vi "ApplyVIPC.vi"   [LabVIEW 2021]
uses:
  <vilib>/Wiresmith Technology/G CLI/CLI Class/CLI.lvclass
  <vilib>/JKI/VIPM API/VIPM API_vipm_api.lvlib
types:
  T1 = enum32{"Invalid", "Standard", "Closed", "Hidden", "Minimized", "Maximized"}
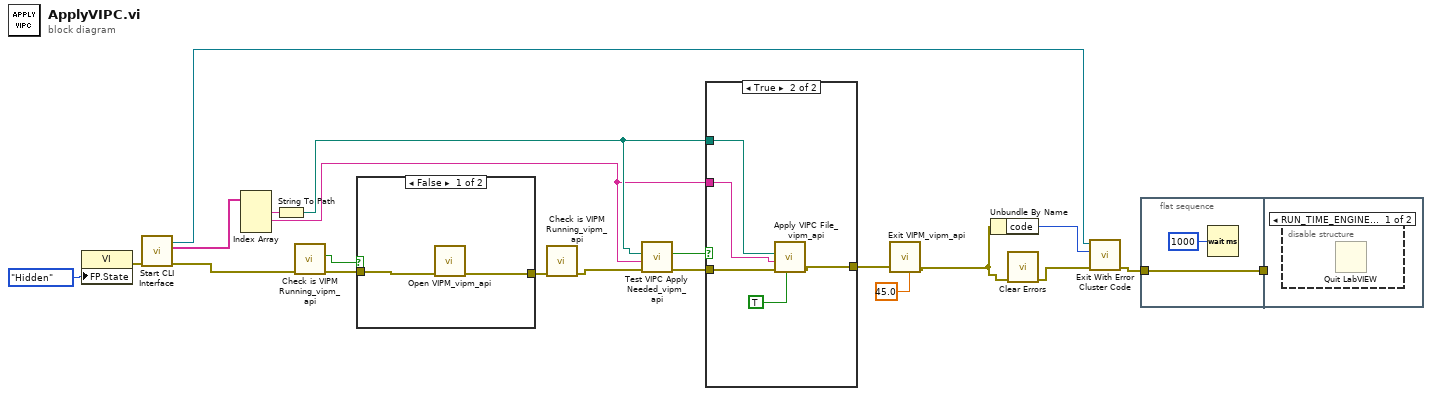
[diagram p0: block diagram]
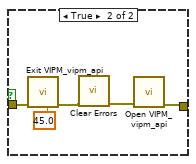
[diagram p2: hidden frame]
diagram:
  n1 = property class="VI"("FP.State"=T1."Hidden" ("Front Panel Window:State")) -> (error out=w20:errorcluster)  [unwired: 2 in, 1 out]
  n2 = call <vilib>:"Start CLI Interface.vi"("error in (no error)"=w20) -> ("error out"=w4:errorcluster, "Custom Parameters"=w18:string[], "CLI out"=w19:refnum<class "CLI.lvclass">)  [unwired: 7 in, 1 out]
  n3 = Index Array(array=w18) -> (element #1=w15:string, element #2=w11:string)  [unwired: 3 in, 1 out]
  n4 = String To Path(string=w15) -> (path=w12:path)
  n5 = call <vilib>:"Check is VIPM Running_vipm_api.vi"("error in (no error)"=w4) -> ("error out"=w10:errorcluster, "is Running"=w9:bool)  [unwired: 9 in]
  n6 = case shown="False" w9 {
    tunnel: w10 -> [w23 w28]
    tunnel: [w22 w24] -> w8
    frame False {
      n7 = call <vilib>:"Open VIPM_vipm_api.vi"("error in (no error)"=w23) -> ("error out"=w22:errorcluster)  [unwired: 10 in]
    }
    frame True {
      n8 = call <vilib>:"Exit VIPM_vipm_api.vi"("Timeout in seconds (0: no timeout)"=45.0, "error in (no error)"=w28) -> ("error out"=w27:errorcluster)  [unwired: 9 in]
      n9 = call <vilib>:"Clear Errors.vi"("error in (no error)"=w27) -> ("error out"=w25:errorcluster)  [unwired: 5 in, 1 out]
      n10 = call <vilib>:"Open VIPM_vipm_api.vi"("error in (no error)"=w25) -> ("error out"=w24:errorcluster)  [unwired: 10 in]
    }
  }
  n11 = call <vilib>:"Check is VIPM Running_vipm_api.vi"("error in (no error)"=w8) -> ("error out"=w5:errorcluster)  [unwired: 9 in, 1 out]
  n12 = call <vilib>:"Test VIPC Apply Needed_vipm_api.vi"("error in (no error)"=w5, "LabVIEW Version (use vipc version)"=w11, "VIPC File Path"=w12) -> ("error out"=w13:errorcluster, "Need to Apply?"=w14:bool)  [unwired: 6 in, 1 out]
  n13 = case shown="True" w14 {
    tunnel: w13 -> [w29 w33]
    tunnel: [w29 w32] -> w6
    tunnel: w12 -> [_ w31]
    tunnel: w11 -> [_ w30]
    frame False {
    }
    frame True {
      n14 = call <vilib>:"Apply VIPC File_vipm_api.vi"("quiet? (T)"=TRUE, "error in (no error)"=w33, "LabVIEW Version"=w30, "VIPC File"=w31) -> ("error out"=w32:errorcluster)  [unwired: 7 in]
    }
  }
  n15 = call <vilib>:"Exit VIPM_vipm_api.vi"("Timeout in seconds (0: no timeout)"=45.0, "error in (no error)"=w6) -> ("error out"=w2:errorcluster)  [unwired: 9 in]
  n16 = Unbundle By Name(w2) -> ("code"=w3:i32)
  n17 = call <vilib>:"Clear Errors.vi"("error in (no error)"=w2) -> ("error out"=w1:errorcluster)  [unwired: 5 in, 1 out]
  n18 = call <vilib>:"Exit With Error Cluster Code.vi"("error in (no error)"=w1, "No Error Code (0)"=w3, "CLI in"=w19) -> ("error out"=w16:errorcluster)  [unwired: 8 in]
  n19 = flat-sequence {
    tunnel: w16 -> [w36]
    tunnel: [w36] -> w17
    tunnel: w17 -> [_]
    frame #0 {
      n20 = Wait (ms)(milliseconds to wait=u32 1000) -> ()  [unwired: 1 out]
    }
    frame #1 {
      n21 = disable-structure shown="RUN_TIME_ENGINE==True" {
        frame condition #0 {
          n22 = Quit LabVIEW() -> ()  [unwired: 1 in]
        }
        frame condition #1 (active) {
        }
      }
    }
  }
